vi "S7Open.vi"(1 "Input":T1={"title"="XXX PLC", "id"=0, "ip"="192.168.10.10", "type"=40, "rack"=0, "slot"=0, "isRunning"=FALSE, "isConnected"=FALSE, "msg"="", "label_status"="STOP", "lable_link"="未连接"} caption="S7PLC" {"type" items=["S7200"=0, "Logo0BA8"=1, "S7200Smart"=2, "S7300"=10, "S7400"=20, "S71200"=30, "S71500"=40]}) -> (0 "Output":T1={"title"="XXX PLC", "id"=0, "ip"="192.168.10.10", "type"=40, "rack"=0, "slot"=0, "isRunning"=FALSE, "isConnected"=FALSE, "msg"="", "label_status"="STOP", "lable_link"="未连接"} caption="S7PLC" {"type" items=["S7200"=0, "Logo0BA8"=1, "S7200Smart"=2, "S7300"=10, "S7400"=20, "S71200"=30, "S71500"=40]})   [LabVIEW 2023]
uses:
  S7Plc.ctl
  D:/Projects/S7View/S7Lib/bin/Debug/S7Lib.dll
  S7Lib/bin/Debug/S7Lib.dll
panel:
  out "Opened":bool
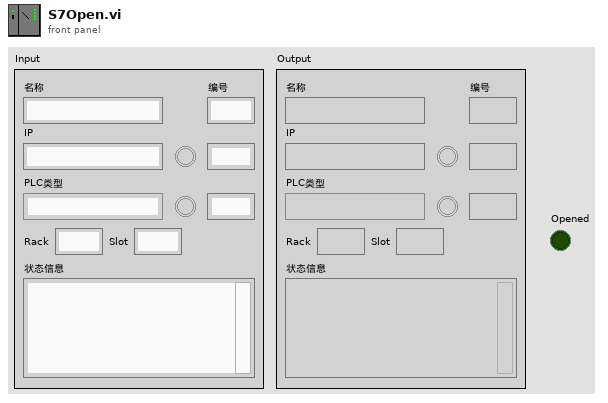
[diagram p1: front panel]
types:
  T1 = typedef "S7Plc.ctl" = cluster{"title":string, "id":i16, "ip":string, "type":i16, "rack":i16, "slot":i16, "isRunning":bool, "isConnected":bool, "msg":string, "label_status":string, "lable_link":string}
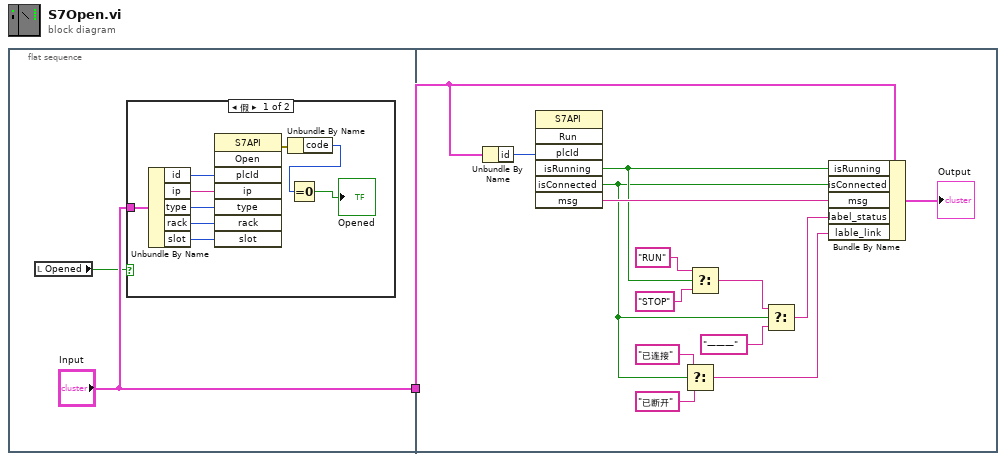
[diagram p0: block diagram]
diagram:
  n1 = flat-sequence {
    tunnel: ["Input"] -> w1
    tunnel: w1 -> [w14]
    frame #0 {
      n2 = local read "Opened"() -> (w2:bool)
      n3 = case shown="假" w2 {
        tunnel: "Input" -> [w7 _]
        frame False {
          n4 = Unbundle By Name(w7) -> ("id"=w8:i16, "ip"=w12:string, "type"=w11:i16, "rack"=w10:i16, "slot"=w9:i16)
          n5 = invoke on="调用节点" class="S7API" method="Open"("plcId"=w8, "ip"=w12, "type"=w11, "rack"=w10, "slot"=w9) -> (error out=w6:errorcluster)  [unwired: 3 in, 7 out]
          n6 = Unbundle By Name(w6) -> ("code"=w5:i32)
          n7 = Equal To 0?(x=w5) -> (x = 0?=→"Opened":bool)
        }
        frame True {
        }
      }
    }
    frame #1 {
      n8 = Unbundle By Name(w14) -> ("id"=w13:i16)
      n9 = invoke on="调用节点" class="S7API" method="Run"("plcId"=w13) -> ("isRunning"=w23:bool, "isConnected"=w22:bool, "msg"=w25:string)  [unwired: 6 in, 4 out]
      n10 = Select(t="已连接", s=w22, f="已断开") -> (s? t:f=w20:string)
      n11 = Select(t="RUN", s=w23, f="STOP") -> (s? t:f=w24:string)
      n12 = Select(t=w24, s=w22, f="———") -> (s? t:f=w21:string)
      n13 = Bundle By Name(cluster=w14, "isRunning"=w23, "isConnected"=w22, "msg"=w25, "label_status"=w21, "lable_link"=w20) -> (→"Output":T1)
    }
  }
